vi "FileName.vi"(11 "String in":string=".tdms") -> (3 "String out":string)   [LabVIEW 2018]
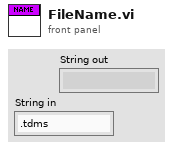
[diagram p1: front panel]
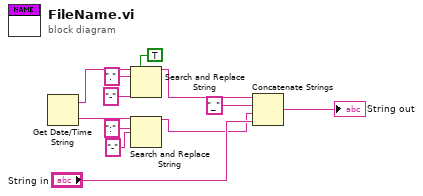
[diagram p0: block diagram]
diagram:
  n1 = Get Date/Time String() -> (date string=w2:string, time string=w5:string)  [unwired: 3 in]
  n2 = Search and Replace String(replace all?=TRUE ("replace all? (F)"), input string=w2, search string=".", replace string="-" ("replace string (\"\")")) -> (result string=w8:string)  [unwired: 4 in, 3 out]
  n3 = Search and Replace String(input string=w5, search string=":", replace string="-" ("replace string (\"\")")) -> (result string=w10:string)  [unwired: 5 in, 3 out]
  n4 = Concatenate Strings(w8, "_" ("string"), w10, "String in") -> (→"String out":string)
